vi "dependency.vi"() -> (3 "clusterzilla":T1)   [LabVIEW 2026, in "dependencies.lvlib"]
uses:
  dependencies.lvlib
  data.ctl
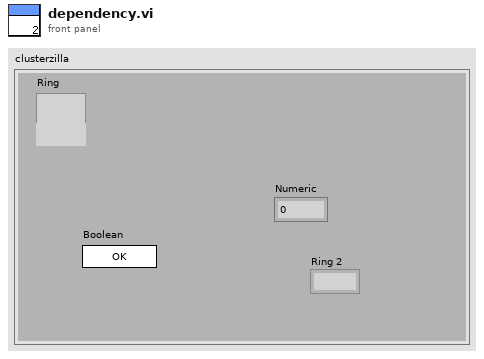
[diagram p1: front panel]
types:
  T1 = typedef "dependencies.lvlib/data.ctl" = cluster{"Ring":u16, "Numeric":dbl, "Boolean":bool, "Ring 2":u16}
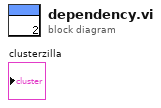
[diagram p0: block diagram]
diagram:
